vi "Air Control View.vi"(11 "Model in":refnum<class "Model.lvclass">) -> ()   [LabVIEW 2016, in "M1M3SupportEUI_Views.lvlib"]
uses:
  M1M3SupportEUI_Views.lvlib
  Model/Model.lvclass
  M1M3 Support Events/M1M3 Support Events.lvclass/M1M3 Support Events.ctl
  SALLV_m1m3/DataTypes/command_TurnAirOn.ctl
  SALLV_m1m3/DataTypes/command_TurnAirOff.ctl
  SALLV_m1m3/DataTypes/command_TestAir.ctl
  SALLV_m1m3/DataTypes/command_TurnLightsOn.ctl
  SALLV_m1m3/DataTypes/command_TurnLightsOff.ctl
  M1M3 Support Events/M1M3 Support Events.lvclass
  SALLV_m1m3/SALLV_m1m3.lvlib
  EUI Events/EUI Events.lvclass
panel:
  out "Lights Status Time Stamp":timestamp
  out "Lights Warning Time Stamp":timestamp
  out "Lights Sensor Mismatch":string
  out "Lights Output Mismatch":string
  out "Any Warning Lights":string
  out "Lights on":string
  out "Lights Output On":string
  out "Lights Commanded On":string
  in  "Turn Lights Off Button":bool
  in  "Turn Lights On Button":bool
  out "Command Sensor Mismatch":string
  out "Command Output Mismatch":string
  out "Any Warning Air":string
  out "Air Valve Closed":string
  out "Air Valve Opened":string
  out "Air Command Output On":string
  out "Air Supply Warning Time Stamp":timestamp
  out "Air Supply Status Time Stamp":timestamp
  in  "Test Air Button":bool
  in  "Turn Air Off Button":bool
  in  "Turn Air On Button":bool
  out "Air Commanded On":string
  # "Air"
  # "Cell Lights"
  # "Commands"
  # "Commands"
  # "Warnings"
  # "Status"
  # "Status"
  # "Warnings"
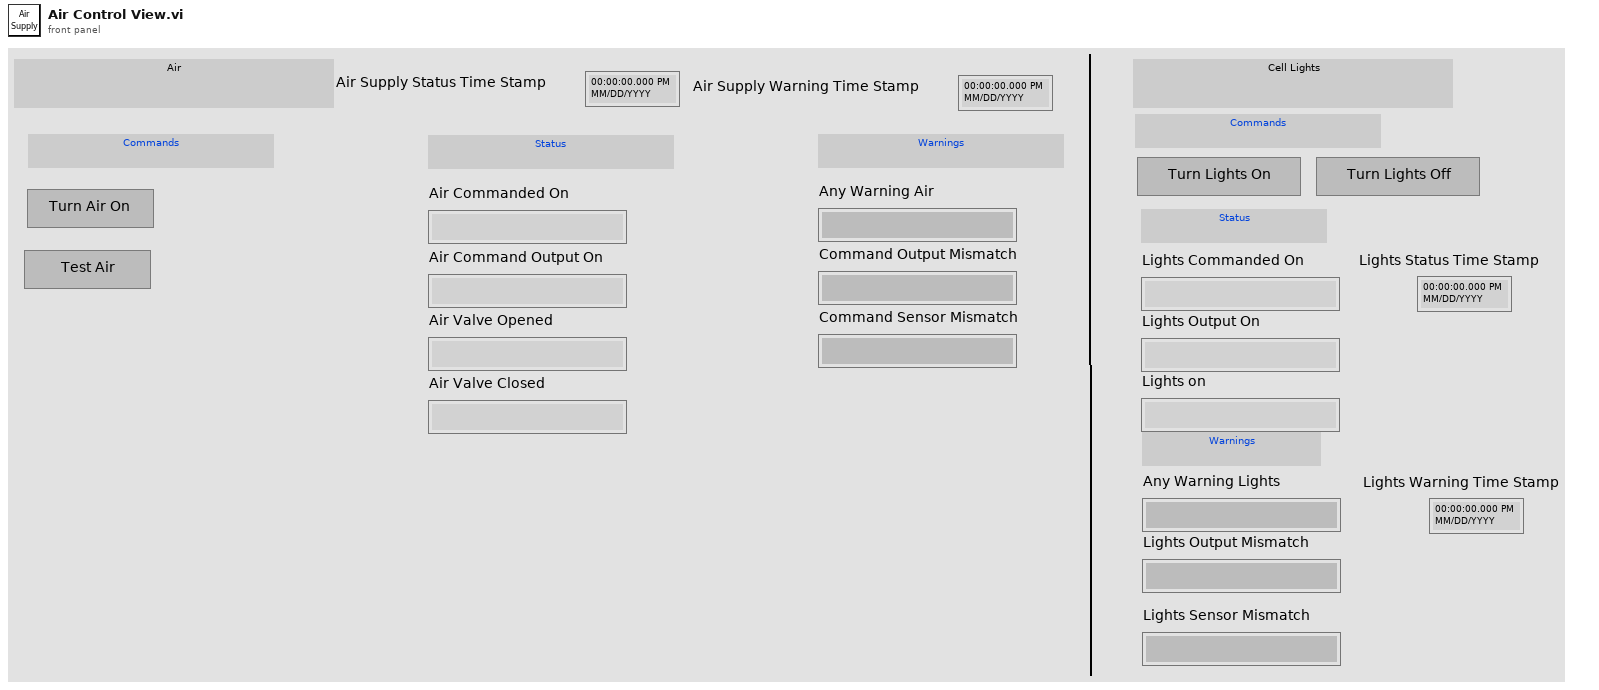
[diagram p1: front panel]
types:
  T1 = typedef "M1M3SupportEUI_TypeDefs.lvlib/M1M3 Support Events.ctl" = cluster{"Inclinometer  Data":refnum<user-event>, "IMS Data":refnum<user-event>, "SAL Connected":refnum<user-event>, "Accelerometer Data":refnum<user-event>, "OuterLoop Data":refnum<user-event>, "ErrorCode Event":refnum<user-event>, "InterlockStatus Event":refnum<user-event>, "InterlockWarning Event":refnum<user-event>, "Gyro Data":refnum<user-event>, "HP Actuator Info Event":refnum<user-event>, " FA Info Event":refnum<user-event>, "HP Monitor Info Event":refnum<user-event>, "FA Data":refnum<user-event>, "HP Actuator data":refnum<user-event>, "HP Monitor data":refnum<user-event>, "Air Supply Status Event":refnum<user-event>, "Air Supply Warning Event":refnum<user-event>, "Power Data":refnum<user-event>, "PID Data":refnum<user-event>, "PID Info Event":refnum<user-event>, "Power Status Event":refnum<user-event>, "Power Supply Status Event":refnum<user-event>, "Power Warning Event":refnum<user-event>, "Summary State Event":refnum<user-event>, "Detailed State Event":refnum<user-event>, "FA Force Warning Event":refnum<user-event>, "FA Warning Event":refnum<user-event>, "FA State Event":refnum<user-event>, "Applied AberrationForces Event":refnum<user-event>, "Applied Acceleration Forcces Event":refnum<user-event>, "Applied Azimuth Forces Event":refnum<user-event>, "Applied Active Optic Forces Event":refnum<user-event>, "Applied Balance Forces Event":refnum<user-event>, "Applied Cylinder Forces Event":refnum<user-event>, "Applied Elevation Forces Event":refnum<user-event>, "Applied Forces Event":refnum<user-event>, "Applied Offset Forces Event":refnum<user-event>, "Applied Static Forces Event":refnum<user-event>, "Applied Thermal Forces Event":refnum<user-event>, "Applied Velocity Forces Event":refnum<user-event>, "Rejected Aberration Force Event":refnum<user-event>, "Rejected Acceleration Forces Event":refnum<user-event>, "Rejected Active Optic Forces Event":refnum<user-event>, "Rejected Azimuth Forces Event":refnum<user-event>, "Rejected Balance Forces Event":refnum<user-event>, "Rejected Cylinder Forces Event":refnum<user-event>, "Rejected Elevation Forces Event":refnum<user-event>, "Rejected Forces Event":refnum<user-event>, "Rejected Offset Forces Event":refnum<user-event>, "Rejected Static Forces Event":refnum<user-event>, "Rejected Thermal Forces Event":refnum<user-event>, "Rejected Velocity Forces Event":refnum<user-event>, "Command Rejection Event":refnum<user-event>, "Setting Verions Event":refnum<user-event>, "Settings Applied Event":refnum<user-event>, "HP Actuator State Event":refnum<user-event>, "HP Actuator Warning Event":refnum<user-event>, "HP Monitor State Event":refnum<user-event>, "HP Monitor Warning Event":refnum<user-event>, "Accelerometer Warning Event":refnum<user-event>, "Applied Settings Match Start Event":refnum<user-event>, "Cell Light Status Event ":refnum<user-event>, "Cell Light Warning Event":refnum<user-event>, "Displacement Sensor Warning Event":refnum<user-event>, "Force Setpoint Warning Event":refnum<user-event>, "Gyro Warning Event ":refnum<user-event>, "ILC Warning Event ":refnum<user-event>, "Inclinometer Sensor Warning Event ":refnum<user-event>}
  T2 = enum16{"", "DetailedState_DetailedStates_DisabledState", "DetailedState_DetailedStates_EnabledState", "DetailedState_DetailedStates_FaultState", "DetailedState_DetailedStates_OfflineState", "DetailedState_DetailedStates_StandbyState", "DetailedState_DetailedStates_ParkedState", "DetailedState_DetailedStates_RaisingState", "DetailedState_DetailedStates_ActiveState", "DetailedState_DetailedStates_LoweringState", "DetailedState_DetailedStates_EngineeringState", "DetailedState_DetailedStates_ParkedEngineeringState", "DetailedState_DetailedStates_RaisingEngineeringState", "DetailedState_DetailedStates_ActiveEngineeringState", "DetailedState_DetailedStates_LoweringEngineeringState", "DetailedState_DetailedStates_LoweringFaultState", "DetailedState_DetailedStates_ProfileHardpointCorrectionState"}
  T3 = typedef "SALLV_m1m3.lvlib/command_TurnAirOn.ctl" = cluster{"TurnAirOn":bool}
  T4 = typedef "SALLV_m1m3.lvlib/command_TurnAirOff.ctl" = cluster{"TurnAirOff":bool}
  T5 = typedef "SALLV_m1m3.lvlib/command_TestAir.ctl" = cluster{"TestAir":bool}
  T6 = typedef "SALLV_m1m3.lvlib/command_TurnLightsOn.ctl" = cluster{"TurnLightsOn":bool}
  T7 = typedef "SALLV_m1m3.lvlib/command_TurnLightsOff.ctl" = cluster{"TurnLightsOff":bool}
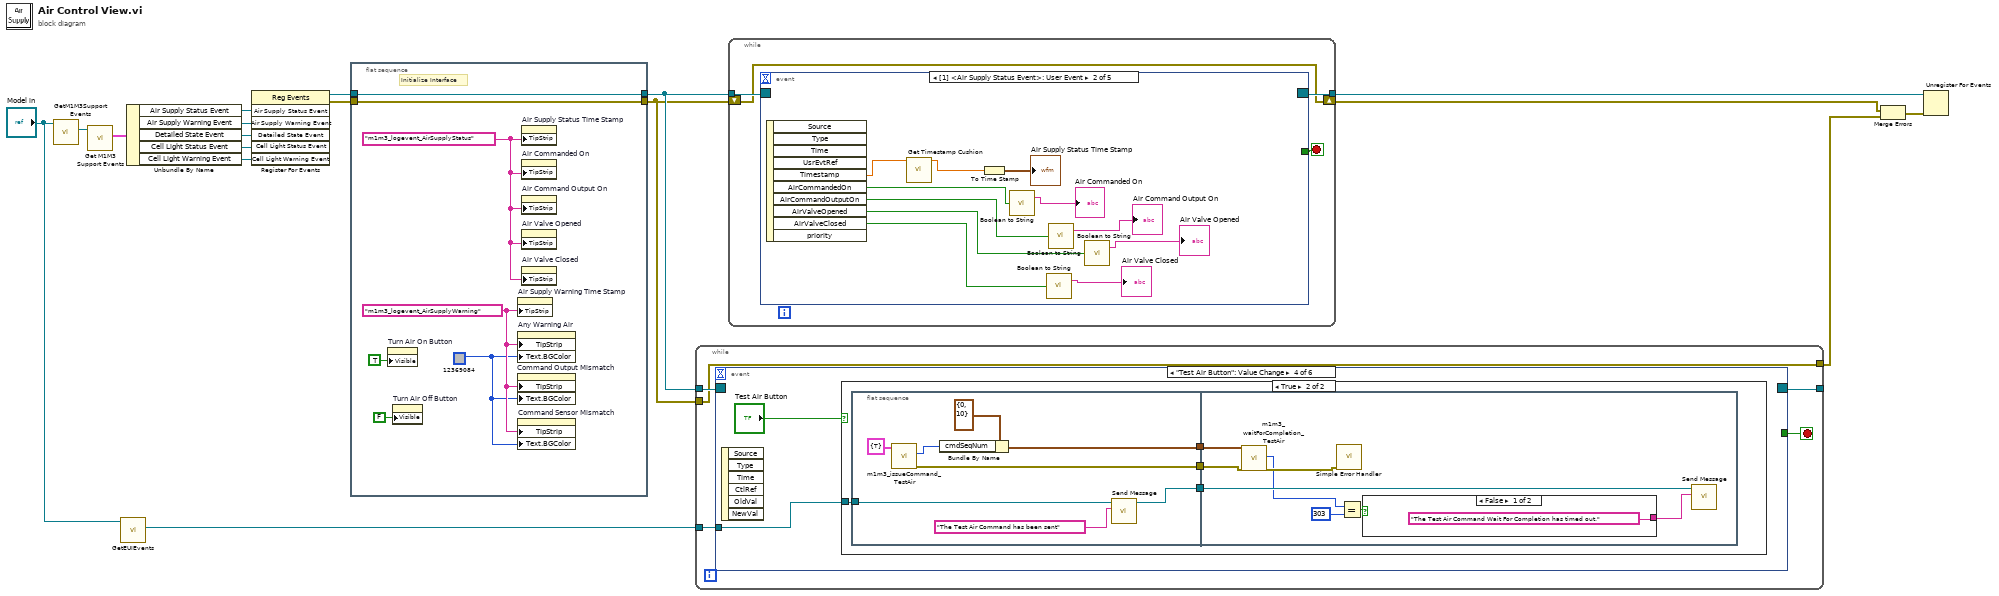
[diagram p0: block diagram]
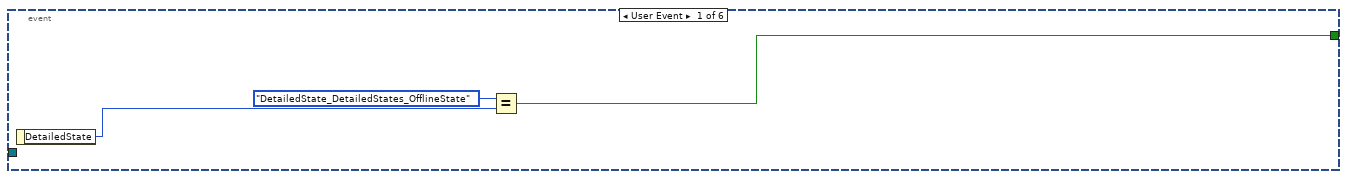
[diagram p2: hidden frame]
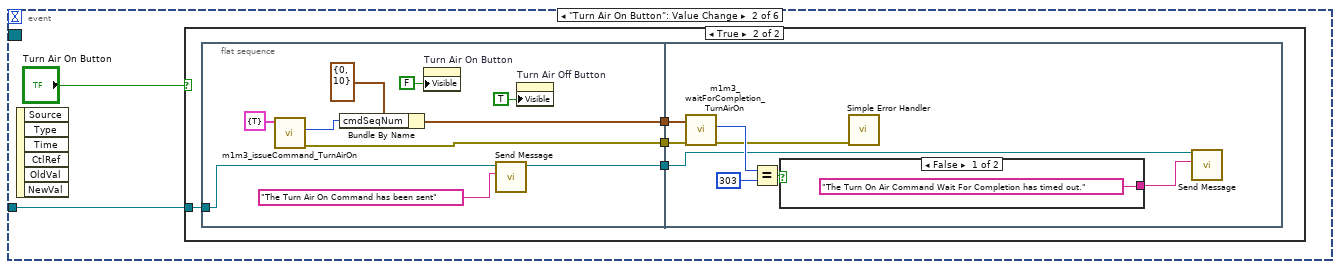
[diagram p3: hidden frame]
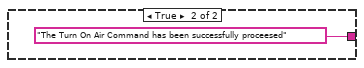
[diagram p5: hidden frame]
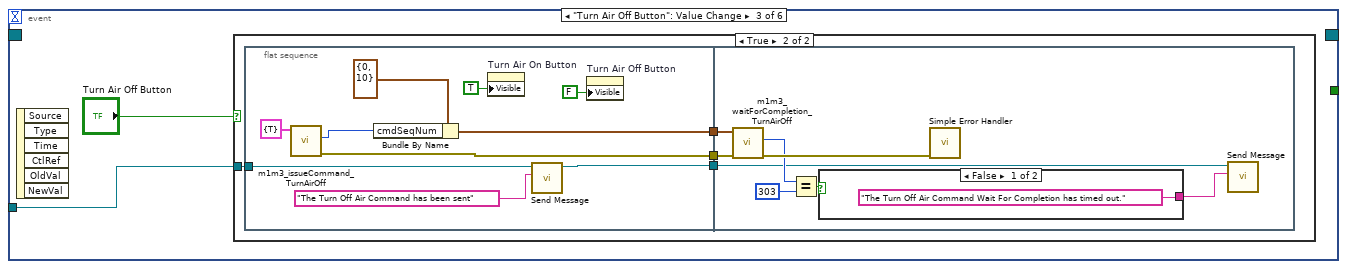
[diagram p6: hidden frame]
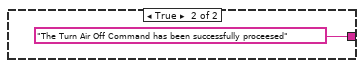
[diagram p8: hidden frame]
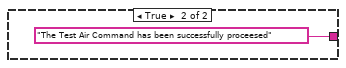
[diagram p10: hidden frame]
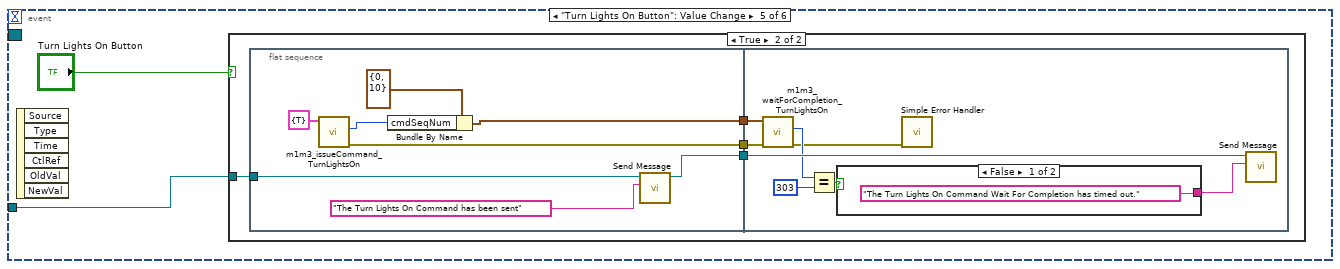
[diagram p11: hidden frame]
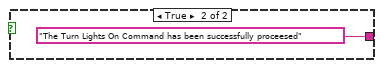
[diagram p13: hidden frame]
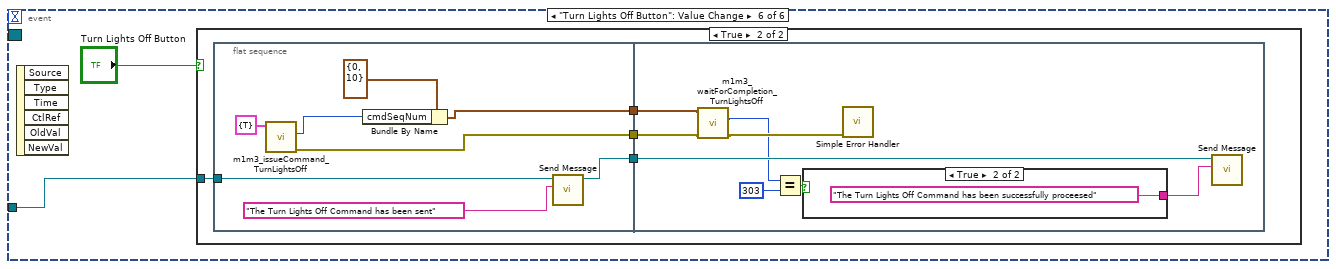
[diagram p14: hidden frame]
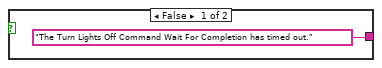
[diagram p16: hidden frame]
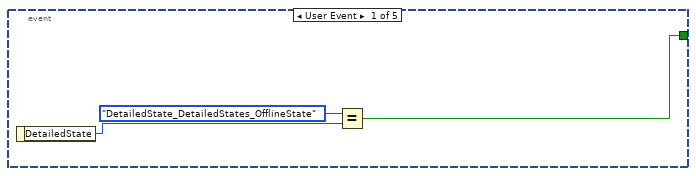
[diagram p17: hidden frame]
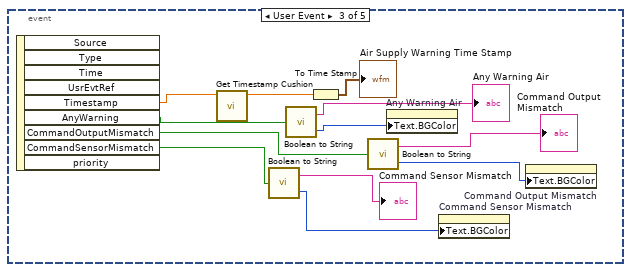
[diagram p18: hidden frame]
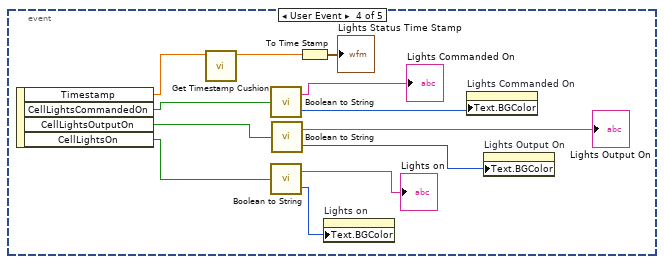
[diagram p19: hidden frame]
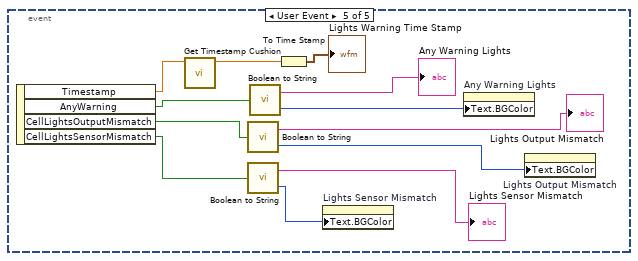
[diagram p20: hidden frame]
diagram:
  n1 = call "GetM1M3SupportEvents.vi"("Model in"="Model in") -> ("M1M3 Support Events out"=w17:refnum<class "M1M3 Support Events.lvclass">)  [unwired: 8 in, 2 out]
  n2 = call "Get M1M3 Support Events.vi"("M1M3 Support Events in"=w17) -> ("M1M3 Support Events"=w16:T1)  [unwired: 9 in, 1 out]
  n3 = call "GetEUIEvents.vi"("Model in"="Model in") -> ("EUI Events out"=w8:refnum<class "EUI Events.lvclass">)  [unwired: 8 in, 2 out]
  n4 = Unbundle By Name(w16) -> ("Air Supply Status Event"=w15:refnum<user-event>, "Air Supply Warning Event"=w14:refnum<user-event>, "Detailed State Event"=w11:refnum<user-event>, "Cell Light Status Event"=w2:refnum<user-event>, "Cell Light Warning Event"=w1:refnum<user-event>)
  n5 = register-events(w15, w14, w11, w2, w1) -> (reference out=w12:refnum<event-registration>, error out=w7:errorcluster)  [unwired: 2 in]
  n6 = flat-sequence {
    tunnel: [w24] -> w10
    tunnel: w12 -> [w24]
    tunnel: w7 -> [w18]
    tunnel: [w18] -> w6
    frame #0 {
      w19 = u32 12369084
      w20 = "m1m3_logevent_AirSupplyWarning" ("Tip Strip")
      w21 = "m1m3_logevent_AirSupplyStatus" ("Tip Strip")
      # "Initialize Interface"
      n7 = property on="Turn Air On Button" class="Bool"("Visible"=TRUE) -> ()  [unwired: 2 in, 2 out]
      n8 = property on="Turn Air Off Button" class="Bool"("Visible"=FALSE) -> ()  [unwired: 2 in, 2 out]
      n9 = property on="Air Supply Warning Time Stamp" class="AbsTime (strict)"("TipStrip"=w20) -> ()  [unwired: 2 in, 2 out]
      n10 = property on="Any Warning Air" class="Str"("TipStrip"=w20, "Text.BGColor"=w19) -> ()  [unwired: 2 in, 2 out]
      n11 = property on="Command Output Mismatch" class="Str"("TipStrip"=w20, "Text.BGColor"=w19) -> ()  [unwired: 2 in, 2 out]
      n12 = property on="Command Sensor Mismatch" class="Str"("TipStrip"=w20, "Text.BGColor"=w19) -> ()  [unwired: 2 in, 2 out]
      n13 = property on="Air Supply Status Time Stamp" class="AbsTime (strict)"("TipStrip"=w21) -> ()  [unwired: 2 in, 2 out]
      n14 = property on="Air Commanded On" class="Str"("TipStrip"=w21) -> ()  [unwired: 2 in, 2 out]
      n15 = property on="Air Command Output On" class="Str"("TipStrip"=w21) -> ()  [unwired: 2 in, 2 out]
      n16 = property on="Air Valve Opened" class="Str"("TipStrip"=w21) -> ()  [unwired: 2 in, 2 out]
      n17 = property on="Air Valve Closed" class="Str"("TipStrip"=w21) -> ()  [unwired: 2 in, 2 out]
    }
  }
  n18 = while {
    tunnel: w10 -> [w29]
    tunnel: [w27] -> _
    tunnel: w8 -> [w26]
    tunnel: w6 -> [w25]
    tunnel: [w25] -> w3
    stop <- w28 stop-if-true
    n19 = event shown="[3] \"Test Air Button\": Value Change" {
      selector: w29 -> [_ _ _ _ _ _]
      dyn-events: [_ _ _ _ _ _] -> w27
      timeout: _ -> [_ _ _ _ _ _]
      tunnel: [w30 _ _ _ _ _] -> w28
      tunnel: w26 -> [_ w33 w59 w85 w109 w133]
      event User Event {
        n20 = event-data() -> ("DetailedState"=w32:T2)  [unwired: 1 in]
        n21 = Equal?(x=T2."DetailedState_DetailedStates_OfflineState", y=w32) -> (x = y?=w30:bool)
      }
      event "Turn Air On Button": Value Change {
        n22 = event-data() -> ()  [unwired: 1 in, 6 out]
        n23 = case shown="True" "Turn Air On Button" {
          tunnel: w33 -> [_ w38]
          frame False {
          }
          frame True {
            n24 = flat-sequence {
              tunnel: w38 -> [w42]
              tunnel: [w41] -> w37
              tunnel: [w40] -> w36
              tunnel: [w39] -> w35
              tunnel: w37 -> [w53]
              tunnel: w36 -> [w52]
              tunnel: w35 -> [w49]
              frame #0 {
                n25 = call "m1m3_issueCommand_TurnAirOn.vi"("command_TurnAirOn_Ctl"=T3 {"TurnAirOn"=TRUE}) -> ("error out"=w40:errorcluster, "function return"=w46:i32)  [unwired: 8 in, 1 out]
                n26 = Bundle By Name(cluster=cluster{"cmdSeqNum":i32, "timeout":u32} {"cmdSeqNum"=0, "timeout"=10} ("waitComplete_Ctl"), "cmdSeqNum"=w46) -> (w41:cluster{"cmdSeqNum":i32, "timeout":u32})
                n27 = property on="Turn Air On Button" class="Bool"("Visible"=FALSE) -> ()  [unwired: 2 in, 2 out]
                n28 = call "Send Message.vi"("Message"="The Turn Air On Command has been sent", "EUI Events in"=w42) -> ("EUI Events out"=w39:refnum<class "EUI Events.lvclass">)  [unwired: 8 in, 1 out]
                n29 = property on="Turn Air Off Button" class="Bool"("Visible"=TRUE) -> ()  [unwired: 2 in, 2 out]
              }
              frame #1 {
                n30 = call "m1m3_waitForCompletion_TurnAirOn.vi"("error in (no error)"=w52, "waitComplete_Ctl"=w53) -> ("error out"=w50:errorcluster, "function return"=w51:i32)  [unwired: 7 in, 1 out]
                n31 = Equal?(x=w51, y=303) -> (x = y?=w55:bool)
                n32 = case shown="False" w55 {
                  tunnel: ["The Turn On Air Command Wait For Completion has timed out." ("Message") "The Turn On Air Command has been successfully proceesed" ("Message")] -> w56
                  frame False {
                  }
                  frame True {
                  }
                }
                n33 = call <vilib>:"Simple Error Handler.vi"("error in (no error)"=w50) -> ()  [unwired: 4 in, 5 out]
                n34 = call "Send Message.vi"("Message"=w56, "EUI Events in"=w49) -> ()  [unwired: 8 in, 2 out]
              }
            }
          }
        }
      }
      event "Turn Air Off Button": Value Change {
        n35 = event-data() -> ()  [unwired: 1 in, 6 out]
        n36 = case shown="True" "Turn Air Off Button" {
          tunnel: w59 -> [_ w62]
          frame False {
          }
          frame True {
            n37 = flat-sequence {
              tunnel: [w68] -> w64
              tunnel: [w67] -> w63
              tunnel: w62 -> [w66]
              tunnel: [w65] -> w61
              tunnel: w64 -> [w82]
              tunnel: w63 -> [w81]
              tunnel: w61 -> [w75]
              frame #0 {
                n38 = call "m1m3_issueCommand_TurnAirOff.vi"("command_TurnAirOff_Ctl"=T4 {"TurnAirOff"=TRUE}) -> ("error out"=w67:errorcluster, "function return"=w72:i32)  [unwired: 8 in, 1 out]
                n39 = Bundle By Name(cluster=cluster{"cmdSeqNum":i32, "timeout":u32} {"cmdSeqNum"=0, "timeout"=10} ("waitComplete_Ctl"), "cmdSeqNum"=w72) -> (w68:cluster{"cmdSeqNum":i32, "timeout":u32})
                n40 = property on="Turn Air On Button" class="Bool"("Visible"=TRUE) -> ()  [unwired: 2 in, 2 out]
                n41 = call "Send Message.vi"("Message"="The Turn Off Air Command has been sent", "EUI Events in"=w66) -> ("EUI Events out"=w65:refnum<class "EUI Events.lvclass">)  [unwired: 8 in, 1 out]
                n42 = property on="Turn Air Off Button" class="Bool"("Visible"=FALSE) -> ()  [unwired: 2 in, 2 out]
              }
              frame #1 {
                n43 = call "m1m3_waitForCompletion_TurnAirOff.vi"("error in (no error)"=w81, "waitComplete_Ctl"=w82) -> ("error out"=w80:errorcluster, "function return"=w76:i32)  [unwired: 7 in, 1 out]
                n44 = Equal?(x=w76, y=303) -> (x = y?=w78:bool)
                n45 = case shown="False" w78 {
                  tunnel: ["The Turn Off Air Command Wait For Completion has timed out." ("Message") "The Turn Air Off Command has been successfully proceesed" ("Message")] -> w79
                  frame False {
                  }
                  frame True {
                  }
                }
                n46 = call <vilib>:"Simple Error Handler.vi"("error in (no error)"=w80) -> ()  [unwired: 4 in, 5 out]
                n47 = call "Send Message.vi"("Message"=w79, "EUI Events in"=w75) -> ()  [unwired: 8 in, 2 out]
              }
            }
          }
        }
      }
      event "Test Air Button": Value Change {
        n48 = event-data() -> ()  [unwired: 1 in, 6 out]
        n49 = case shown="True" "Test Air Button" {
          tunnel: w85 -> [_ w90]
          frame False {
          }
          frame True {
            n50 = flat-sequence {
              tunnel: w90 -> [w94]
              tunnel: [w93] -> w89
              tunnel: [w92] -> w88
              tunnel: [w91] -> w87
              tunnel: w89 -> [w103]
              tunnel: w88 -> [w102]
              tunnel: w87 -> [w101]
              frame #0 {
                n51 = call "m1m3_issueCommand_TestAir.vi"("command_TestAir_Ctl"=T5 {"TestAir"=TRUE}) -> ("error out"=w91:errorcluster, "function return"=w96:i32)  [unwired: 8 in, 1 out]
                n52 = Bundle By Name(cluster=cluster{"cmdSeqNum":i32, "timeout":u32} {"cmdSeqNum"=0, "timeout"=10} ("waitComplete_Ctl"), "cmdSeqNum"=w96) -> (w92:cluster{"cmdSeqNum":i32, "timeout":u32})
                n53 = call "Send Message.vi"("Message"="The Test Air Command has been sent", "EUI Events in"=w94) -> ("EUI Events out"=w93:refnum<class "EUI Events.lvclass">)  [unwired: 8 in, 1 out]
              }
              frame #1 {
                n54 = call "m1m3_waitForCompletion_TestAir.vi"("error in (no error)"=w101, "waitComplete_Ctl"=w102) -> ("error out"=w100:errorcluster, "function return"=w99:i32)  [unwired: 7 in, 1 out]
                n55 = call <vilib>:"Simple Error Handler.vi"("error in (no error)"=w100) -> ()  [unwired: 4 in, 5 out]
                n56 = Equal?(x=w99, y=303) -> (x = y?=w105:bool)
                n57 = case shown="False" w105 {
                  tunnel: ["The Test Air Command Wait For Completion has timed out." ("Message") "The Test Air Command has been successfully proceesed" ("Message")] -> w106
                  frame False {
                  }
                  frame True {
                  }
                }
                n58 = call "Send Message.vi"("Message"=w106, "EUI Events in"=w103) -> ()  [unwired: 8 in, 2 out]
              }
            }
          }
        }
      }
      event "Turn Lights On Button": Value Change {
        n59 = event-data() -> ()  [unwired: 1 in, 6 out]
        n60 = case shown="True" "Turn Lights On Button" {
          tunnel: w109 -> [_ w114]
          frame False {
          }
          frame True {
            n61 = flat-sequence {
              tunnel: w114 -> [w121]
              tunnel: [w120] -> w113
              tunnel: [w116] -> w112
              tunnel: [w115] -> w111
              tunnel: w113 -> [w127]
              tunnel: w112 -> [w126]
              tunnel: w111 -> [w125]
              frame #0 {
                n62 = call "m1m3_issueCommand_TurnLightsOn.vi"("command_TurnLightsOn_Ctl"=T6 {"TurnLightsOn"=TRUE}) -> ("error out"=w116:errorcluster, "function return"=w117:i32)  [unwired: 8 in, 1 out]
                n63 = Bundle By Name(cluster=cluster{"cmdSeqNum":i32, "timeout":u32} {"cmdSeqNum"=0, "timeout"=10} ("waitComplete_Ctl"), "cmdSeqNum"=w117) -> (w115:cluster{"cmdSeqNum":i32, "timeout":u32})
                n64 = call "Send Message.vi"("Message"="The Turn Lights On Command has been sent", "EUI Events in"=w121) -> ("EUI Events out"=w120:refnum<class "EUI Events.lvclass">)  [unwired: 8 in, 1 out]
              }
              frame #1 {
                n65 = call "m1m3_waitForCompletion_TurnLightsOn.vi"("error in (no error)"=w126, "waitComplete_Ctl"=w125) -> ("error out"=w123:errorcluster, "function return"=w124:i32)  [unwired: 7 in, 1 out]
                n66 = Equal?(x=w124, y=303) -> (x = y?=w129:bool)
                n67 = case shown="False" w129 {
                  tunnel: ["The Turn Lights On Command Wait For Completion has timed out." ("Message") "The Turn Lights On Command has been successfully proceesed" ("Message")] -> w130
                  frame False {
                  }
                  frame True {
                  }
                }
                n68 = call <vilib>:"Simple Error Handler.vi"("error in (no error)"=w123) -> ()  [unwired: 4 in, 5 out]
                n69 = call "Send Message.vi"("Message"=w130, "EUI Events in"=w127) -> ()  [unwired: 8 in, 2 out]
              }
            }
          }
        }
      }
      event "Turn Lights Off Button": Value Change {
        n70 = event-data() -> ()  [unwired: 1 in, 6 out]
        n71 = case shown="True" "Turn Lights Off Button" {
          tunnel: w133 -> [_ w138]
          frame False {
          }
          frame True {
            n72 = flat-sequence {
              tunnel: w138 -> [w145]
              tunnel: [w144] -> w137
              tunnel: [w140] -> w136
              tunnel: [w139] -> w135
              tunnel: w137 -> [w151]
              tunnel: w136 -> [w149]
              tunnel: w135 -> [w150]
              frame #0 {
                n73 = call "m1m3_issueCommand_TurnLightsOff.vi"("command_TurnLightsOff_Ctl"=T7 {"TurnLightsOff"=TRUE}) -> ("error out"=w140:errorcluster, "function return"=w142:i32)  [unwired: 8 in, 1 out]
                n74 = Bundle By Name(cluster=cluster{"cmdSeqNum":i32, "timeout":u32} {"cmdSeqNum"=0, "timeout"=10} ("waitComplete_Ctl"), "cmdSeqNum"=w142) -> (w139:cluster{"cmdSeqNum":i32, "timeout":u32})
                n75 = call "Send Message.vi"("Message"="The Turn Lights Off Command has been sent", "EUI Events in"=w145) -> ("EUI Events out"=w144:refnum<class "EUI Events.lvclass">)  [unwired: 8 in, 1 out]
              }
              frame #1 {
                n76 = call "m1m3_waitForCompletion_TurnLightsOff.vi"("error in (no error)"=w149, "waitComplete_Ctl"=w150) -> ("error out"=w148:errorcluster, "function return"=w147:i32)  [unwired: 7 in, 1 out]
                n77 = Equal?(x=w147, y=303) -> (x = y?=w153:bool)
                n78 = case shown="True" w153 {
                  tunnel: ["The Turn Lights Off Command Wait For Completion has timed out." ("Message") "The Turn Lights Off Command has been successfully proceesed" ("Message")] -> w154
                  frame False {
                  }
                  frame True {
                  }
                }
                n79 = call <vilib>:"Simple Error Handler.vi"("error in (no error)"=w148) -> ()  [unwired: 4 in, 5 out]
                n80 = call "Send Message.vi"("Message"=w154, "EUI Events in"=w151) -> ()  [unwired: 8 in, 2 out]
              }
            }
          }
        }
      }
    }
  }
  n81 = while {
    tunnel: w10 -> [w160]
    tunnel: [w159] -> w13
    shift-right: [w157] -> w4
    shift-left: w6 -> [w157]
    stop <- w158 stop-if-true
    n82 = event shown="[1] <Air Supply Status Event>: User Event" {
      selector: w160 -> [_ _ _ _ _]
      dyn-events: [_ _ _ _ _] -> w159
      timeout: _ -> [_ _ _ _ _]
      tunnel: [w161 _ _ _ _] -> w158
      event User Event {
        n83 = event-data() -> ("DetailedState"=w163:T2)  [unwired: 1 in]
        n84 = Equal?(x=T2."DetailedState_DetailedStates_OfflineState", y=w163) -> (x = y?=w161:bool)
      }
      event User Event {
        n85 = event-data() -> ("Timestamp"=w164:dbl, "AirCommandedOn"=w172:bool, "AirCommandOutputOn"=w170:bool, "AirValveOpened"=w168:bool, "AirValveClosed"=w166:bool)  [unwired: 1 in, 5 out]
        n86 = call "Get Timestamp Cushion.vi"("DoubleTimestampRepresentation"=w164) -> ("TimestampCushion"=w174:dbl)  [unwired: 10 in]
        n87 = To Time Stamp(1:w174) -> (0:→"Air Supply Status Time Stamp":timestamp)
        n88 = call "Boolean to String.vi"("BooleanValue"=w172) -> ("StringForm"=→"Air Commanded On":string)  [unwired: 1 out]
        n89 = call "Boolean to String.vi"("BooleanValue"=w166) -> ("StringForm"=→"Air Valve Closed":string)  [unwired: 1 out]
        n90 = call "Boolean to String.vi"("BooleanValue"=w170) -> ("StringForm"=→"Air Command Output On":string)  [unwired: 1 out]
        n91 = call "Boolean to String.vi"("BooleanValue"=w168) -> ("StringForm"=→"Air Valve Opened":string)  [unwired: 1 out]
      }
      event User Event {
        n92 = event-data() -> ("Timestamp"=w175:dbl, "AnyWarning"=w184:bool, "CommandOutputMismatch"=w182:bool, "CommandSensorMismatch"=w180:bool)  [unwired: 1 in, 5 out]
        n93 = call "Get Timestamp Cushion.vi"("DoubleTimestampRepresentation"=w175) -> ("TimestampCushion"=w186:dbl)  [unwired: 10 in]
        n94 = call "Boolean to String.vi"("BooleanValue"=w180) -> ("StringForm"=→"Command Sensor Mismatch":string, "BackgroundColor"=w176:u32)
        n95 = call "Boolean to String.vi"("BooleanValue"=w184) -> ("StringForm"=→"Any Warning Air":string, "BackgroundColor"=w178:u32)
        n96 = To Time Stamp(1:w186) -> (0:→"Air Supply Warning Time Stamp":timestamp)
        n97 = call "Boolean to String.vi"("BooleanValue"=w182) -> ("StringForm"=→"Command Output Mismatch":string, "BackgroundColor"=w177:u32)
        n98 = property on="Any Warning Air" class="Str"("Text.BGColor"=w178) -> ()  [unwired: 2 in, 2 out]
        n99 = property on="Command Sensor Mismatch" class="Str"("Text.BGColor"=w176) -> ()  [unwired: 2 in, 2 out]
        n100 = property on="Command Output Mismatch" class="Str"("Text.BGColor"=w177) -> ()  [unwired: 2 in, 2 out]
      }
      event User Event {
        n101 = event-data() -> ("Timestamp"=w197:dbl, "CellLightsCommandedOn"=w195:bool, "CellLightsOutputOn"=w193:bool, "CellLightsOn"=w192:bool)  [unwired: 1 in]
        n102 = call "Get Timestamp Cushion.vi"("DoubleTimestampRepresentation"=w197) -> ("TimestampCushion"=w198:dbl)  [unwired: 10 in]
        n103 = call "Boolean to String.vi"("BooleanValue"=w195) -> ("StringForm"=→"Lights Commanded On":string, "BackgroundColor"=w189:u32)
        n104 = call "Boolean to String.vi"("BooleanValue"=w192) -> ("StringForm"=→"Lights on":string, "BackgroundColor"=w187:u32)
        n105 = call "Boolean to String.vi"("BooleanValue"=w193) -> ("StringForm"=→"Lights Output On":string, "BackgroundColor"=w188:u32)
        n106 = To Time Stamp(1:w198) -> (0:→"Lights Status Time Stamp":timestamp)
        n107 = property on="Lights on" class="Str"("Text.BGColor"=w187) -> ()  [unwired: 2 in, 2 out]
        n108 = property on="Lights Commanded On" class="Str"("Text.BGColor"=w189) -> ()  [unwired: 2 in, 2 out]
        n109 = property on="Lights Output On" class="Str"("Text.BGColor"=w188) -> ()  [unwired: 2 in, 2 out]
      }
      event User Event {
        n110 = event-data() -> ("Timestamp"=w209:dbl, "AnyWarning"=w207:bool, "CellLightsOutputMismatch"=w206:bool, "CellLightsSensorMismatch"=w205:bool)  [unwired: 1 in]
        n111 = call "Get Timestamp Cushion.vi"("DoubleTimestampRepresentation"=w209) -> ("TimestampCushion"=w210:dbl)  [unwired: 10 in]
        n112 = call "Boolean to String.vi"("BooleanValue"=w206) -> ("StringForm"=→"Lights Output Mismatch":string, "BackgroundColor"=w200:u32)
        n113 = call "Boolean to String.vi"("BooleanValue"=w205) -> ("StringForm"=→"Lights Sensor Mismatch":string, "BackgroundColor"=w199:u32)
        n114 = call "Boolean to String.vi"("BooleanValue"=w207) -> ("StringForm"=→"Any Warning Lights":string, "BackgroundColor"=w201:u32)
        n115 = To Time Stamp(1:w210) -> (0:→"Lights Warning Time Stamp":timestamp)
        n116 = property on="Lights Sensor Mismatch" class="Str"("Text.BGColor"=w199) -> ()  [unwired: 2 in, 2 out]
        n117 = property on="Any Warning Lights" class="Str"("Text.BGColor"=w201) -> ()  [unwired: 2 in, 2 out]
        n118 = property on="Lights Output Mismatch" class="Str"("Text.BGColor"=w200) -> ()  [unwired: 2 in, 2 out]
      }
    }
  }
  n119 = Merge Errors(w4, w3) -> (w5:errorcluster)
  n120 = Unregister For Events(event registration refnum=w13, error in=w5) -> ()  [unwired: 1 out]
